vi "读取模板.vi"(11 "Filename":path=path "D:/Desktop/test.lvm" caption="文件名") -> (1 "模板特征参数 2":dbl[][](array[numeric]))   [LabVIEW 2018]
panel:
  out "error out":errorcluster caption="错误输出"
  out "Filename Out":path caption="文件名输出"
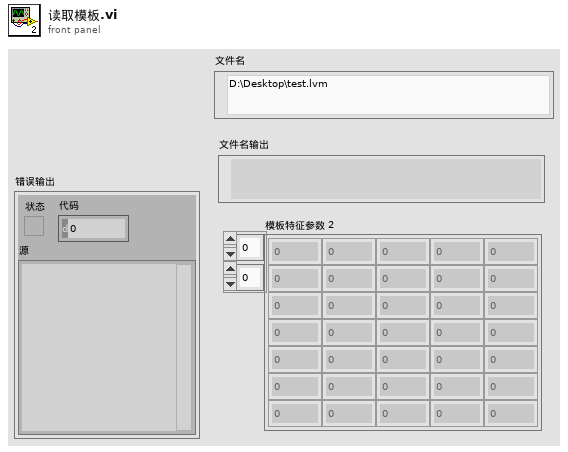
[diagram p1: front panel]
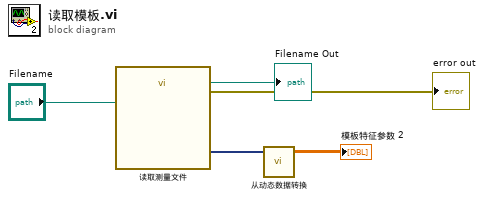
[diagram p0: block diagram]
diagram:
  n1 = call "读取测量文件"("Filename"="Filename") -> ("error out"=→"error out":errorcluster, "Filename Out"=→"Filename Out":path, "Signals"=w5:dynamicdata)  [unwired: 5 in, 3 out]
  n2 = call "从动态数据转换"("Dynamic Data Type"=w5) -> ("Array"=→"模板特征参数 2":dbl[][])  [unwired: 3 in]
